vi "Test_InsertRemoveItems.vi"(8 "error in (no error)":errorcluster, 11 "TestCase in":refnum<class "ListImp_Functional.lvclass">) -> (0 "error out":errorcluster, 3 "TestCase out":refnum<class "ListImp_Functional.lvclass">)   [LabVIEW 2009, in "ListImp_Functional.lvclass"]
uses:
  ListImp_Functional.lvclass
  ListImp_Functional.lvclass/ListImp_Functional.ctl
  source/Lists/List/List.lvclass
  source/Lists.Interfaces/String/String.lvclass
  UnitTestComparisons/UnitTestComparisons.lvlib
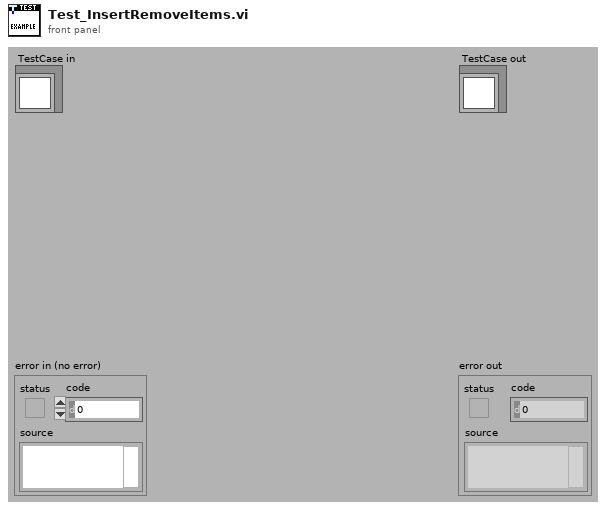
[diagram p1: front panel]
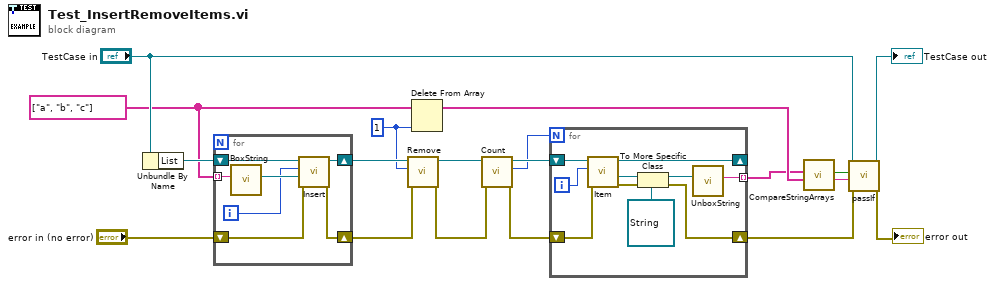
[diagram p0: block diagram]
diagram:
  w11 = 1 ("Index")
  w12 = string[] ["a", "b", "c"]
  n1 = Unbundle By Name("TestCase in") -> ("List"=w16:refnum<class "List.lvclass">)
  n2 = for {
    tunnel: w12 -> [w23] mode=indexing
    shift-right: [w25] -> w14
    shift-left: w16 -> [w26]
    shift-right: [w20] -> w13
    shift-left: "error in (no error)" -> [w21]
    i -> [w22]
    n3 = call "BoxString.vi"("String"=w23) -> ("String out"=w24:refnum<class "String.lvclass">)  [unwired: 10 in]
    n4 = call-dynamic "Insert.vi"("error in (no error)"=w21, "Item"=w24, "Index"=w22, "List in"=w26) -> ("error out"=w20:errorcluster, "List out"=w25:refnum<class "List.lvclass">)  [unwired: 6 in]
  }
  n5 = call-dynamic "Remove.vi"("error in (no error)"=w13, "Index"=w11, "List in"=w14) -> ("error out"=w6:errorcluster, "List out"=w9:refnum<class "List.lvclass">)  [unwired: 6 in, 1 out]
  n6 = Delete From Array(array=w12, index=w11) -> (array with subset deleted=w2:string[])  [unwired: 1 in, 1 out]
  n7 = call-dynamic "Count.vi"("error in (no error)"=w6, "List in"=w9) -> ("error out"=w5:errorcluster, "Number of Items"=w7:i32, "List out"=w8:refnum<class "List.lvclass">)  [unwired: 7 in]
  n8 = for {
    N: w7 -> [_]
    shift-right: [w35] -> _
    shift-left: w8 -> [w36]
    shift-right: [w28] -> w10
    shift-left: w5 -> [w34]
    tunnel: [w27] -> w1 mode=indexing
    i -> [w33]
    n9 = call-dynamic "Item.vi"("error in (no error)"=w34, "Index"=w33, "List in"=w36) -> ("error out"=w31:errorcluster, "Item"=w32:refnum<class>, "List out"=w35:refnum<class "List.lvclass">)  [unwired: 6 in]
    n10 = To More Specific Class(target class=refnum<class "String.lvclass"> refnum ("LapDog.Collections.v0.Lists.Interfaces.lvlib:String.lvclass"), reference=w32, error in=w31) -> (specific class reference=w29:refnum<class "String.lvclass">, error out=w28:errorcluster)
    n11 = call "UnboxString.vi"("String in"=w29) -> ("String"=w27:string)  [unwired: 10 in]
  }
  n12 = call "CompareStringArrays.vi"("Expected Strings"=w2, "Actual Strings"=w1) -> ("Message"=w3:string, "Equal?"=w4:bool)  [unwired: 8 in]
  n13 = call-dynamic "passIf.vi"("error in (no error)"=w10, "message (\"\")"=w3, "pass"=w4, "TestCase in"="TestCase in") -> ("error out"=→"error out":errorcluster, "TestCase out"=→"TestCase out":refnum<class "ListImp_Functional.lvclass">)  [unwired: 6 in]
